vi "Test.vi"(8 "error in (no error)":errorcluster, 11 "FTP in":refnum<class "FTP.lvclass">) -> (0 "error out":errorcluster)   [LabVIEW 2017, in "FTP_UpgradeCSMF.lvlib" / "FTP.lvclass"]
uses:
  FTP.lvclass
  controls/Dir-File Info.ctl
  controls/Dir-File Type.ctl
panel:
  out "Dir-File Info Array 2":T1[](array[typedef])
  out "Slide":u8(slide) scale=0.0..100.0
  out "Dir-File Info Array":T1[](array[typedef])
  out "time stamp":timestamp
  out "FileSize":i64
  out "cmdStrings":string
  in  "Local FilePath":path=path "C:/Users/jgoldberg.EVALUMATION/Desktop/adcConv.m"
  out "Current Directory":string
  in  "passWord":string
  in  "userName":string
  in  "address":string
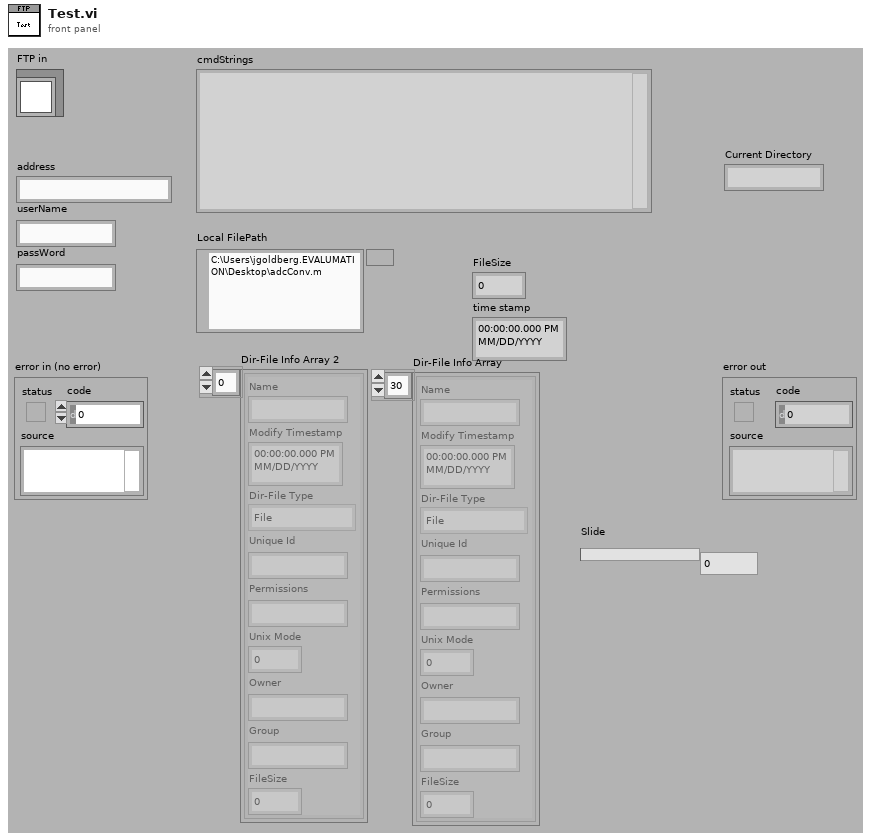
[diagram p1: front panel]
types:
  T1 = typedef "FTP_UpgradeCSMF.lvlib/FTP.lvclass/Dir-File Info.ctl" = cluster{"Name":string, "Modify Timestamp":timestamp, "Dir-File Type":T2, "Unique Id":string, "Permissions":string, "Unix Mode":u16, "Owner":string, "Group":string, "FileSize":i64}
  T2 = typedef "FTP_UpgradeCSMF.lvlib/FTP.lvclass/Dir-File Type.ctl" = enum16{"File", "Listed Directory", "Parent Directory", "Directory", "Unknown"}
  T3 = typedef "CmdCluster.ctl" = cluster{"CmdSting":string, "FromClient":bool}
  T4 = typedef "FTP.lvclass/File Transfer Status.ctl" = cluster{"File Name":string, "Percent Complete":u8, "File Size (in bytes)":i64, "Bytes Sent or Rcvd":i64}
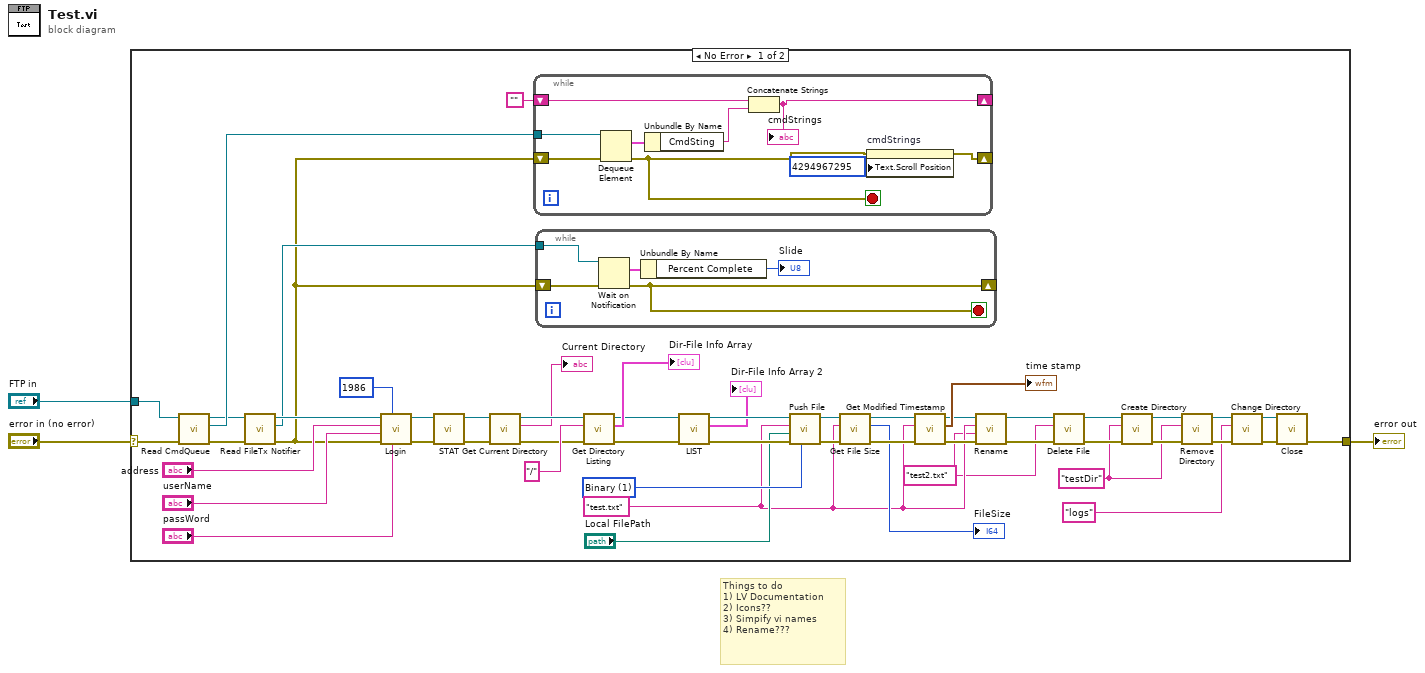
[diagram p0: block diagram]
diagram:
  # "Things to do\n1) LV Documentation\n2) Icons??\n3) Simpify vi names\n4) Rename???"
  n1 = case shown="No Error" "error in (no error)" {
    selector: "error in (no error)" -> [w25 w70]
    tunnel: [w55 w70] -> w2
    tunnel: "FTP in" -> [w24 _]
    frame No Error {
      w11 = "test2.txt" ("New FileName")
      w44 = "testDir" ("Remote Directory")
      w36 = u16 1 items=["ASCII", "Binary"] ("Type")
      w12 = "test.txt" ("FileName")
      n2 = call "Read CmdQueue.vi"("error in (no error)"=w25, "FTP in"=w24) -> ("error out"=w21:errorcluster, "CmdQueue"=w51:refnum<queue>, "FTP out"=w22:refnum<class "FTP.lvclass">)  [unwired: 7 in]
      n3 = call "Read FileTx Notifier.vi"("error in (no error)"=w21, "FTP in"=w22) -> ("error out"=w17:errorcluster, "FileTx Notifier"=w18:refnum<notifier>, "FTP out"=w20:refnum<class "FTP.lvclass">)  [unwired: 7 in]
      n4 = call "Login.vi"("passWord"="passWord", "remote port (21)"=u16 1986, "error in (no error)"=w17, "userName"="userName", "address"="address", "FTP in"=w20) -> ("error out"=w19:errorcluster, "FTP out"=w23:refnum<class "FTP.lvclass">)  [unwired: 4 in]
      n5 = call "STAT.vi"("error in (no error)"=w19, "FTP in"=w23) -> ("error out"=w28:errorcluster, "FTP out"=w29:refnum<class "FTP.lvclass">)  [unwired: 7 in, 1 out]
      n6 = call "Get Current Directory.vi"("error in (no error)"=w28, "FTP in"=w29) -> ("error out"=w41:errorcluster, "Current Directory"=→"Current Directory":string, "FTP out"=w42:refnum<class "FTP.lvclass">)  [unwired: 7 in]
      n7 = while {
        tunnel: w51 -> [w69]
        shift-right: [w62] -> _
        shift-left: w17 -> [w68]
        shift-right: [w64] -> _
        shift-left: "" -> [w66]
        stop <- w61 stop-if-true
        n8 = Dequeue Element(queue=w69, error in (no error)=w68) -> (element=w67:T3, error out=w61:errorcluster)  [unwired: 1 in, 2 out]
        n9 = Unbundle By Name(w67) -> ("CmdSting"=w65:string)
        n10 = Concatenate Strings(w66, w65) -> (w64:string)
        "cmdStrings" <- w64
        n11 = property on="cmdStrings" class="Str"(error in=w61, "Text.Scroll Position"=u32 4294967295) -> (error out=w62:errorcluster)  [unwired: 1 in, 1 out]
      }
      n12 = while {
        tunnel: w18 -> [w59]
        shift-right: [w56] -> _
        shift-left: w17 -> [w60]
        stop <- w56 stop-if-true
        n13 = Wait on Notification(notifier=w59, error in (no error)=w60) -> (notification=w58:T4, error out=w56:errorcluster)  [unwired: 2 in, 2 out]
        n14 = Unbundle By Name(w58) -> ("Percent Complete"=→"Slide":u8)
      }
      n15 = call "Get Directory Listing.vi"("error in (no error)"=w41, "RemoteDirectory"="/", "FTP in"=w42) -> ("error out"=w26:errorcluster, "Dir-File Info Array"=→"Dir-File Info Array":T1[], "FTP out"=w27:refnum<class "FTP.lvclass">)  [unwired: 6 in]
      n16 = call "LIST.vi"("error in (no error)"=w26, "FTP in"=w27) -> ("error out"=w38:errorcluster, "Dir-File Info Array"=→"Dir-File Info Array 2":T1[], "FTP out"=w37:refnum<class "FTP.lvclass">)  [unwired: 7 in]
      n17 = call "Push File.vi"("Type (Binary)"=w36, "error in (no error)"=w38, "Local FilePath"="Local FilePath", "Remote FileName"=w12, "FTP in"=w37) -> ("error out"=w33:errorcluster, "FTP out"=w34:refnum<class "FTP.lvclass">)  [unwired: 5 in]
      n18 = call "Get File Size.vi"("error in (no error)"=w33, "Remote FileName"=w12, "FTP in"=w34) -> ("error out"=w31:errorcluster, "FileSize"=→"FileSize":i64, "FTP out"=w32:refnum<class "FTP.lvclass">)  [unwired: 6 in]
      n19 = call "Get Modified Timestamp.vi"("error in (no error)"=w31, "RemoteFileName"=w12, "FTP in"=w32) -> ("error out"=w16:errorcluster, "Modified Timestamp"=→"time stamp":timestamp, "FTP out"=w15:refnum<class "FTP.lvclass">)  [unwired: 6 in]
      n20 = call "Rename.vi"("error in (no error)"=w16, "New FileName"=w11, "File To Rename"=w12, "FTP in"=w15) -> ("error out"=w13:errorcluster, "FTP out"=w14:refnum<class "FTP.lvclass">)  [unwired: 6 in]
      n21 = call "Delete File.vi"("error in (no error)"=w13, "RemoteFileName"=w11, "FTP in"=w14) -> ("error out"=w48:errorcluster, "FTP out"=w47:refnum<class "FTP.lvclass">)  [unwired: 7 in]
      n22 = call "Create Directory.vi"("error in (no error)"=w48, "Remote Directory"=w44, "FTP in"=w47) -> ("error out"=w45:errorcluster, "FTP out"=w46:refnum<class "FTP.lvclass">)  [unwired: 7 in]
      n23 = call "Remove Directory.vi"("error in (no error)"=w45, "Remote Directory"=w44, "FTP in"=w46) -> ("error out"=w9:errorcluster, "FTP out"=w10:refnum<class "FTP.lvclass">)  [unwired: 7 in]
      n24 = call "Change Directory.vi"("error in (no error)"=w9, "RemoteDirectory"="logs" ("Remote Directory"), "FTP in"=w10) -> ("error out"=w7:errorcluster, "FTP out"=w8:refnum<class "FTP.lvclass">)  [unwired: 7 in]
      n25 = call "Close.vi"("error in (no error)"=w7, "FTP in"=w8) -> ("error out"=w55:errorcluster)  [unwired: 9 in]
    }
    frame Error {
    }
  }
  "error out" <- w2
